vi "Set Debugger.vi"(8 "error in (no error)":errorcluster, 10 "Debuger":T1, 11 "CO2 Actor in":refnum<class "CO2 Actor.lvclass">) -> (0 "error out":errorcluster, 3 "CO2 Actor out":refnum<class "CO2 Actor.lvclass">)   [LabVIEW 2015, in "cRIO-Carbondioxide.lvlib" / "CO2-Actor.lvlib" / "CO2 Actor.lvclass"]
uses:
  CO2 Actor.lvclass
  cRIO-CO2/Debugger.ctl
  CO2 Actor.lvclass/CO2 Actor.ctl
  cRIO-CO2/cRIO-CO2.lvclass
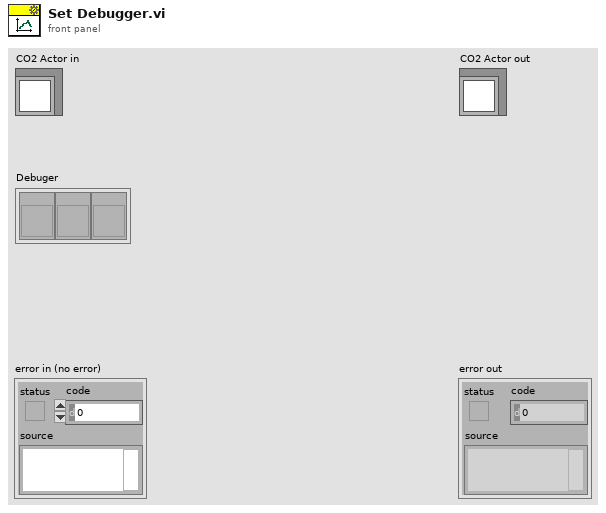
[diagram p1: front panel]
types:
  T1 = typedef "cRIO-Carbondioxide.lvlib/cRIO-CO2.lvlib/cRIO-CO2.lvclass/Debugger.ctl" = cluster{"Log Ref":refnum<vi>, "Debugger Graph Chart Ref":refnum<vi>, "Debug Rng Ref":refnum<vi>}
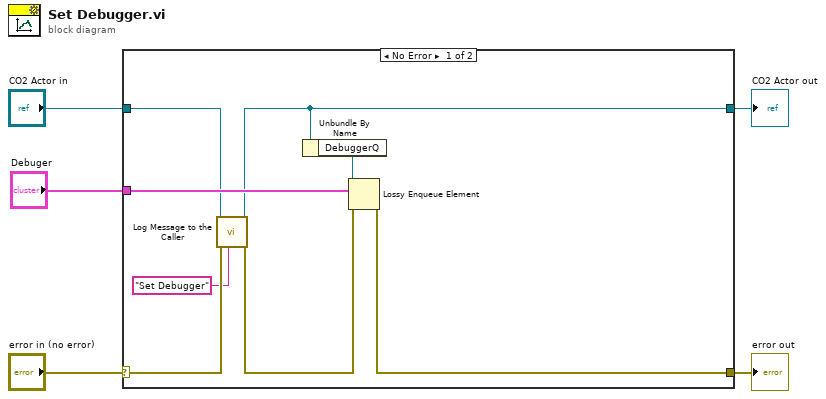
[diagram p0: block diagram]
diagram:
  n1 = case shown="No Error" "error in (no error)" {
    selector: "error in (no error)" -> [w8 w15]
    tunnel: [w12 w15] -> w4
    tunnel: [w9 w14] -> w2
    tunnel: "CO2 Actor in" -> [w10 w14]
    tunnel: "Debuger" -> [w11 _]
    frame No Error {
      n2 = call-dynamic "Log Message to the Caller.vi"("String (\"\" = no message to send)"="Set Debugger" ("String (\"OK\")"), "error in (no error)"=w8, "CO2 Actor in"=w10) -> ("error out"=w7:errorcluster, "CO2 Actor out"=w9:refnum<class "CO2 Actor.lvclass">)  [unwired: 7 in]
      n3 = Unbundle By Name(w9) -> ("DebuggerQ"=w13:refnum<queue>)
      n4 = Lossy Enqueue Element(queue=w13, element=w11, error in (no error)=w7) -> (error out=w12:errorcluster)  [unwired: 3 out]
    }
    frame Error {
    }
  }
  "error out" <- w4
  "CO2 Actor out" <- w2
